vi "convertDataDIO64.vi"(8 "error in (no error)":errorcluster, 10 "Data":T1={"Timestamps ms"=[0.0, 0.005, 0.009, 0.012], "Bitmap"=[[TRUE, FALSE, FALSE, FALSE, FALSE, FALSE, FALSE, FALSE, FALSE, TRUE, TRUE, FALSE, FALSE, FALSE, FALSE, FALSE], [FALSE, FALSE, FALSE, FALSE, FALSE, FALSE, FALSE, FALSE, FALSE, FALSE, FALSE, FALSE, FALSE, FALSE, FALSE, TRUE], [FALSE, FALSE, FALSE, FALSE, TRUE, FALSE, FALSE, FALSE, FALSE, FALSE, FALSE, FALSE, FALSE, FALSE, FALSE, FALSE]]} {"Timestamps ms" format="%.6f"}, 11 "DIO64Output in":refnum<class "DIO64Output.lvclass">) -> (0 "error out":errorcluster, 1 "#ports":u8=1 min=1 max=8, 2 "data":u16[][](array[numeric])=[[1]] format="%x", 3 "DIO64Output out":refnum<class "DIO64Output.lvclass">, 5 "mask":u16[](array[numeric])=[1] format="%.0x")   [LabVIEW 2009, in "Hardware.lvlib" / "Channels.lvlib" / "DIO64Output.lvclass"]
uses:
  DIO64Output.lvclass
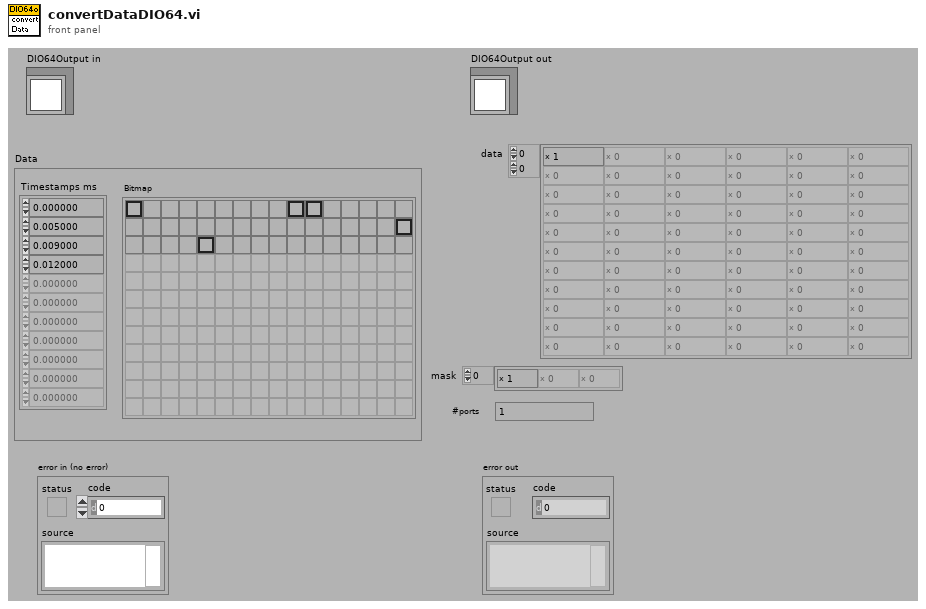
[diagram p1: front panel]
types:
  T1 = cluster{"Timestamps ms":dbl[], "Bitmap":bool[][]}
  T2 = cluster{"Master Clock source":string, "Master Clock rate":dbl, "Start trigger line":string, "Scan rate":dbl, "Stop trigger line":string, "Sample Number":dbl}
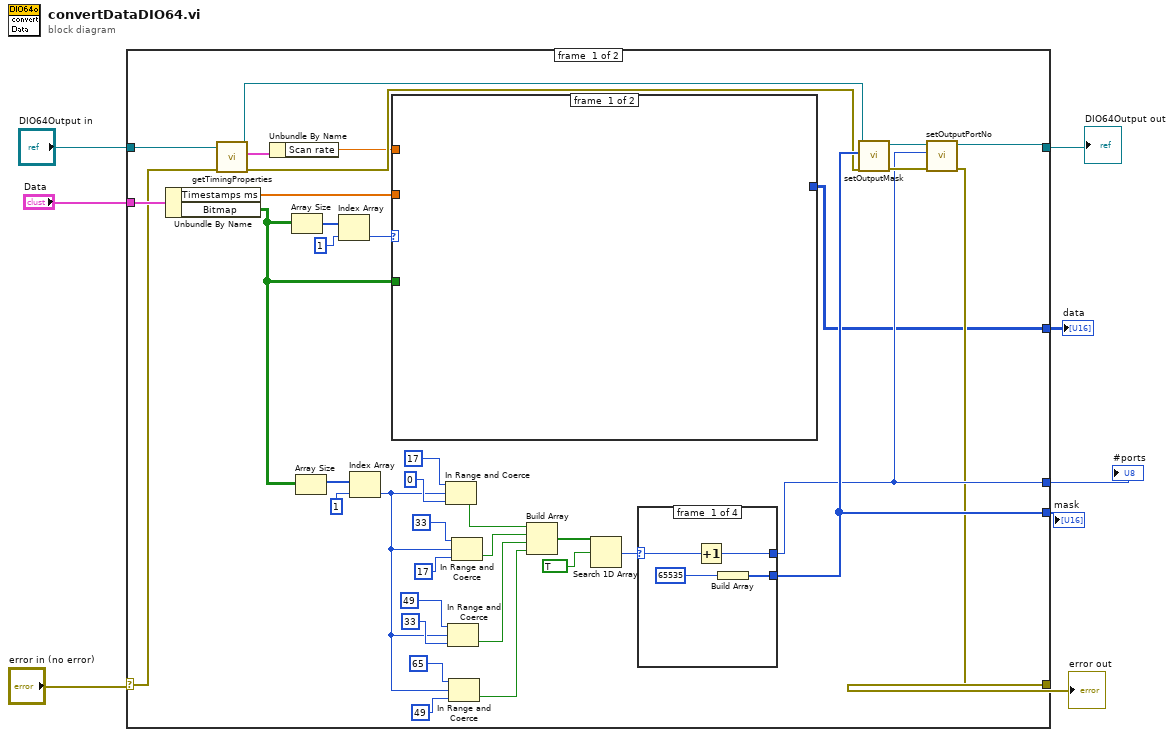
[diagram p0: block diagram]
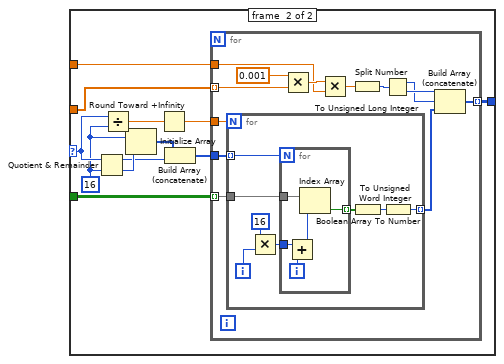
[diagram p2: hidden frame]
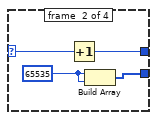
[diagram p3: hidden frame]
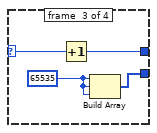
[diagram p4: hidden frame]
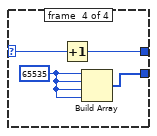
[diagram p5: hidden frame]
diagram:
  n1 = case shown="No Error" "error in (no error)" {
    selector: "error in (no error)" -> [w42 w101]
    tunnel: [w16 w101] -> w7
    tunnel: [w18 w100] -> w5
    tunnel: "DIO64Output in" -> [w44 w100]
    tunnel: [w10 _] -> w4
    tunnel: "Data" -> [w45 _]
    tunnel: [w22 _] -> w2
    tunnel: [w19 _] -> w1
    frame #0 {
      n2 = Unbundle By Name(w45) -> ("Timestamps ms"=w14:dbl[], "Bitmap"=w9:bool[][])
      n3 = call-dynamic "getTimingProperties.vi"("error in (no error)"=w42, "DigitalOutput.lvclass in"=w44) -> ("error out"=w17:errorcluster, "Timing"=w43:T2, "DigitalOutput.lvclass out"=w23:refnum<class "DIO64Output.lvclass">)  [unwired: 7 in]
      n4 = Unbundle By Name(w43) -> ("Scan rate"=w15:dbl)
      n5 = Array Size(array=w9) -> (size(s)=w13:i32[])
      n6 = Array Size(array=w9) -> (size(s)=w41:i32[])
      n7 = Index Array(array=w13, index=1) -> (element=w11:i32)
      n8 = Index Array(array=w41, index=1) -> (element=w31:i32)
      n9 = case shown="1..64" w11 {
        selector: w11 -> [_ w54]
        tunnel: w9 -> [_ w55]
        tunnel: w14 -> [_ w48]
        tunnel: [_ w47] -> w10
        tunnel: w15 -> [_ w46]
        frame #0 {
        }
        frame #1 {
          w52 = 16 ("y")
          n10 = Quotient & Remainder(x=w54, y=w52) -> (x-y*floor(x/y)=w50:i32, floor(x/y)=w53:i32)
          n11 = Divide(x=w54, y=w52) -> (x/y=w57:dbl)
          n12 = Initialize Array(w52, w53) -> (w51:i32[])
          n13 = Round Toward +Infinity(x=w57) -> (ceil(x): smallest int >= x=w56:dbl)
          n14 = Build Array (concatenate)(w51, w50) -> (w49:i32[])
          n15 = for {
            tunnel: w56 -> [w70]
            tunnel: w55 -> [w69] mode=indexing
            tunnel: w49 -> [w68]
            tunnel: w48 -> [w64] mode=indexing
            tunnel: w46 -> [w63]
            tunnel: [w59] -> w47 mode=indexing
            n16 = for {
              N: w70 -> [_]
              tunnel: w69 -> [w71]
              tunnel: [w74] -> w60 mode=indexing
              tunnel: w68 -> [w72] mode=indexing
              i -> [w78]
              n17 = Multiply(x=16, y=w78) -> (x*y=w77:i32)
              n18 = for {
                N: w72 -> [_]
                tunnel: w71 -> [w81]
                tunnel: w77 -> [w83]
                tunnel: [w79] -> w73 mode=indexing
                i -> [w82]
                n19 = Add(x=w83, y=w82) -> (x+y=w80:i32)
                n20 = Index Array(array=w81, index=w80) -> (element=w79:bool)
              }
              n21 = Boolean Array To Number(Boolean array=w73) -> (number=w75:u32)
              n22 = To Unsigned Word Integer(number=w75) -> (unsigned 16bit integer=w74:u16)
            }
            n23 = Multiply(x=0.001, y=w64) -> (x*y=w67:dbl)
            n24 = Multiply(x=w67, y=w63) -> (x*y=w66:dbl)
            n25 = To Unsigned Long Integer(number=w66) -> (unsigned 32bit integer=w65:u32)
            n26 = Split Number(x=w65) -> (hi(x)=w61:u16, lo(x)=w62:u16)
            n27 = Build Array (concatenate)(w62, w61, w60) -> (w59:u16[])
          }
        }
      }
      n28 = In Range and Coerce(upper limit=17, x=w31, lower limit=0) -> (In Range?=w30:bool)  [unwired: 1 out]
      n29 = In Range and Coerce(upper limit=49, x=w31, lower limit=33) -> (In Range?=w28:bool)  [unwired: 1 out]
      n30 = In Range and Coerce(upper limit=65, x=w31, lower limit=49) -> (In Range?=w27:bool)  [unwired: 1 out]
      n31 = In Range and Coerce(upper limit=33, x=w31, lower limit=17) -> (In Range?=w29:bool)  [unwired: 1 out]
      n32 = Build Array(w30, w29, w28, w27) -> (w26:bool[])
      n33 = Search 1D Array(1D array=w26, element=TRUE) -> (index of element=w24:i32)  [unwired: 1 in]
      n34 = case shown="0, Default" w24 {
        selector: w24 -> [w85 w89 w93 w97]
        tunnel: [w86 w90 w94 w98] -> w22
        tunnel: [w84 w88 w92 w96] -> w19
        frame #0 {
          n35 = Increment(x=w85) -> (x+1=w84:i32)
          n36 = Build Array(u16 65535) -> (w86:u16[])
        }
        frame #1 {
          w91 = u16 65535
          n37 = Increment(x=w89) -> (x+1=w88:i32)
          n38 = Build Array(w91, w91) -> (w90:u16[])
        }
        frame #2 {
          w95 = u16 65535
          n39 = Increment(x=w93) -> (x+1=w92:i32)
          n40 = Build Array(w95, w95, w95) -> (w94:u16[])
        }
        frame #3 {
          w99 = u16 65535
          n41 = Increment(x=w97) -> (x+1=w96:i32)
          n42 = Build Array(w99, w99, w99, w99) -> (w98:u16[])
        }
      }
      n43 = call "setOutputMask.vi"("error in (no error)"=w17, "mask"=w22, "DIO64Output.lvclass in"=w23) -> ("error out"=w20:errorcluster, "DIO64Output.lvclass out"=w21:refnum<class "DIO64Output.lvclass">)  [unwired: 7 in]
      n44 = call "setOutputPortNo.vi"("error in (no error)"=w20, "#ports"=w19, "DIO64Output.lvclass in"=w21) -> ("error out"=w16:errorcluster, "DIO64Output.lvclass out"=w18:refnum<class "DIO64Output.lvclass">)  [unwired: 7 in]
    }
    frame #1 {
    }
  }
  "error out" <- w7
  "DIO64Output out" <- w5
  "data" <- w4
  "#ports" <- w1
  "mask" <- w2
